vi "ConvertBoolToFWDREV.vi"(1 "Bool In":bool) -> (0 "Direction Out":u8)   [LabVIEW 2014]
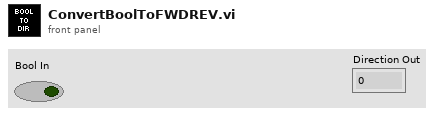
[diagram p1: front panel]
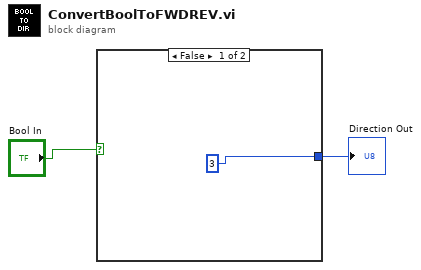
[diagram p0: block diagram]
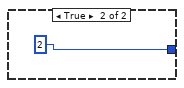
[diagram p2: hidden frame]
diagram:
  n1 = case shown="False" "Bool In" {
    tunnel: [3 2] -> w1
    frame False {
    }
    frame True {
    }
  }
  "Direction Out" <- w1
